vi "Open Core FP.vi"(8 "error in (no error)":errorcluster, 11 "Log in":refnum<class "Log.lvclass">) -> (0 "error out":errorcluster, 3 "Log out":refnum<class "Log.lvclass">)   [LabVIEW 2015, in "AMS UI.lvlib" / "Log.lvclass"]
uses:
  Log.lvclass
  AMS Gas Actor/AMS Gas Actor.lvclass/AMS Gas Actor.ctl
  AMS Gas Actor/AMS Gas Actor.lvclass
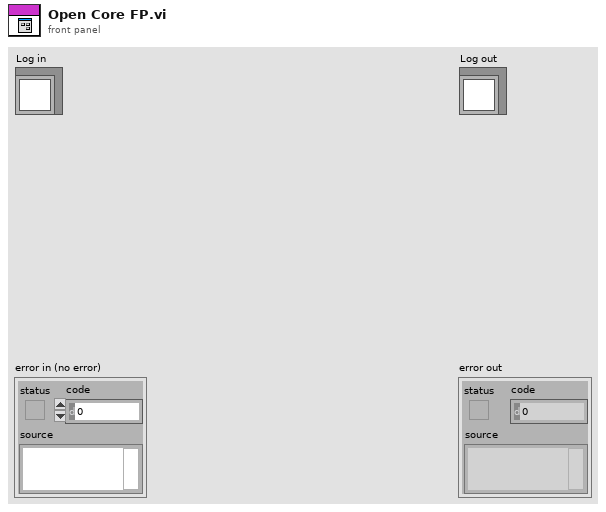
[diagram p1: front panel]
types:
  T1 = enum32{"Invalid", "Standard", "Closed", "Hidden", "Minimized", "Maximized"}
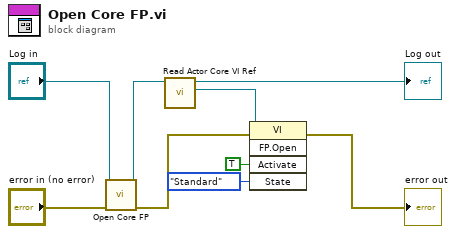
[diagram p0: block diagram]
diagram:
  n1 = call-parent "Open Core FP.vi"("error in (no error)"="error in (no error)", "AMS Gas Actor in"="Log in") -> ("error out"=w2:errorcluster, "AMS Gas Actor out"=w7:refnum<class "Log.lvclass">)  [unwired: 8 in]
  n2 = call "Read Actor Core VI Ref.vi"("AMS Gas Actor in"=w7) -> ("Actor Core VI Ref"=w5:refnum<vi>, "AMS Gas Actor out"=→"Log out":refnum<class "Log.lvclass">)  [unwired: 9 in]
  n3 = invoke class="VI" method="FP.Open"(reference=w5, error in=w2, "Activate"=TRUE ("Activate?"), "State"=T1."Standard") -> (error out=→"error out":errorcluster)  [unwired: 1 in, 4 out]
